vi "AppendWaveToFile.vi"(6 "Waveform":u16[](array[numeric]), 8 "error in (no error)":errorcluster, 10 "Append?":bool, 11 "HDF5 Dataset Ref":T1) -> (0 "error out":errorcluster, 2 "Elements Added?":bool, 3 "HDF5 Dataset out":T1)   [LabVIEW 2020]
uses:
  <vilib>/UPVI/lvhdf5/library.llb/HDF5 Ref.ctl
  <vilib>/UPVI/lvhdf5/dataset.llb/Append Element(s) to Dataset (Variant).vi
  <vilib>/UPVI/lvhdf5/dataset.llb/Append Element(s) to Dataset.xnode
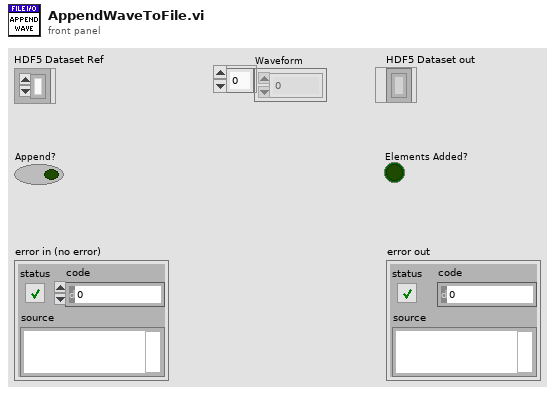
[diagram p1: front panel]
types:
  T1 = typedef "HDF5 Ref.ctl" = refnum<k1>
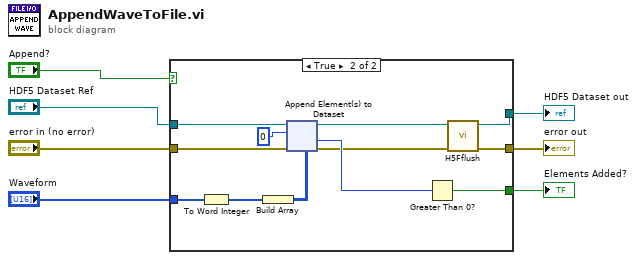
[diagram p0: block diagram]
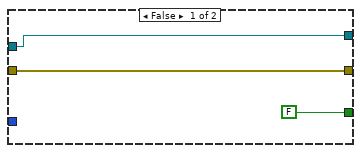
[diagram p2: hidden frame]
diagram:
  n1 = case shown="True" "Append?" {
    tunnel: "HDF5 Dataset Ref" -> [w10 w20]
    tunnel: "error in (no error)" -> [w9 w19]
    tunnel: [w10 w12] -> w5
    tunnel: [w9 w13] -> w4
    tunnel: "Waveform" -> [_ w18]
    tunnel: [FALSE w15] -> w1
    frame False {
    }
    frame True {
      n2 = To Word Integer(number=w18) -> (16bit integer=w17:i16[])
      n3 = Build Array(w17) -> (w21:i16[][])
      n4 = xnode "Append Element(s) to Dataset"("Dimension to Extend (0)"=0, "HDF5 Dataset Ref"=w20, "error in (no error)"=w19, "Data Element(s)"=w21) -> ("HDF5 Dataset out"=w11:T1, "Number of Elements Added"=w16:i32, "error out"=w14:errorcluster)  [unwired: 1 out]
      n5 = Greater Than 0?(x=w16) -> (x > 0?=w15:bool)
      n6 = call <vilib>:"H5Fflush.vi"("error in (no error)"=w14, "HDF5 Ref"=w11) -> ("error out"=w13:errorcluster, "HDF5 Ref out"=w12:T1)  [unwired: 6 in]
    }
  }
  "HDF5 Dataset out" <- w5
  "error out" <- w4
  "Elements Added?" <- w1
